vi "ShortcutToFile.vi"(8 "error in (no error)":errorcluster, 10 "write? (F)":bool, 11 "Shortcut file":path) -> (0 "error out":errorcluster, 2 "succeeded?":bool, 3 "Shortcut file out":path)   [LabVIEW 2015]
doc: "This will return a list of items in a folder that are shortcuts (*.lnk). The Path to the Shortcut and the path to item pointed to by the Shortcut are included.\n\nExample:\n Location of Shortcuts: C:\\My Documents\\Misc\n\n Output:\n PATH TO SHORCUT: C:\\My Documents\\Misc\\RF Gain.doc.lnk\n PATH TO ITEM: I:\\Engineers\\John Smith\\RF Gain.doc\n\n PATH TO SHORCUT: C:\\My Documents\\Misc\\Schedule.mpp.lnk\n PATH TO ITEM: I:\\Projects\\ATE\\Planning\\Schedule.mpp\n\n\nReferences:\n Windows Shell - http://msdn.microsoft.com/en-us/library/bb773177(v=VS.85).aspx\n Shell Object - http://msdn.microsoft.com/en-us/library/bb774094(v=VS.85).aspx\n ShellLinkObject Object - http://msdn.microsoft.com/en-us/library/bb774004(v=VS.85).aspx\n\n Changing the icon of EXE files programatically - http://social.msdn.microsoft.com/forums/en-US/csharpgeneral/thread/9e23a82c-8bed-4b96-8b9a-4c2b6136a622/"
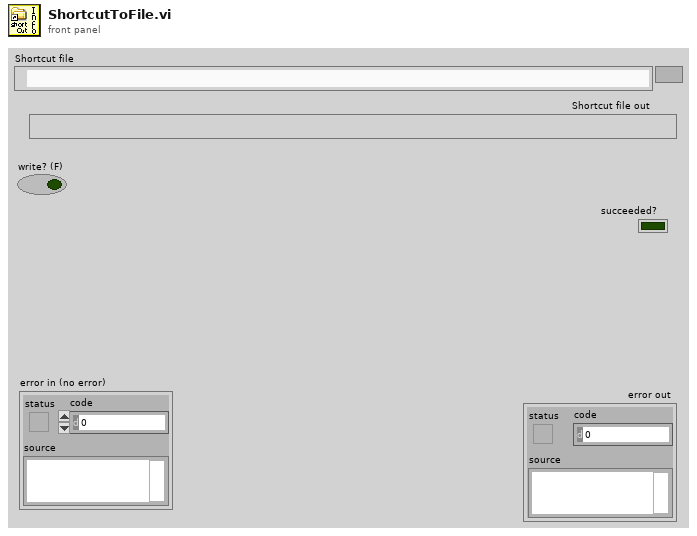
[diagram p1: front panel]
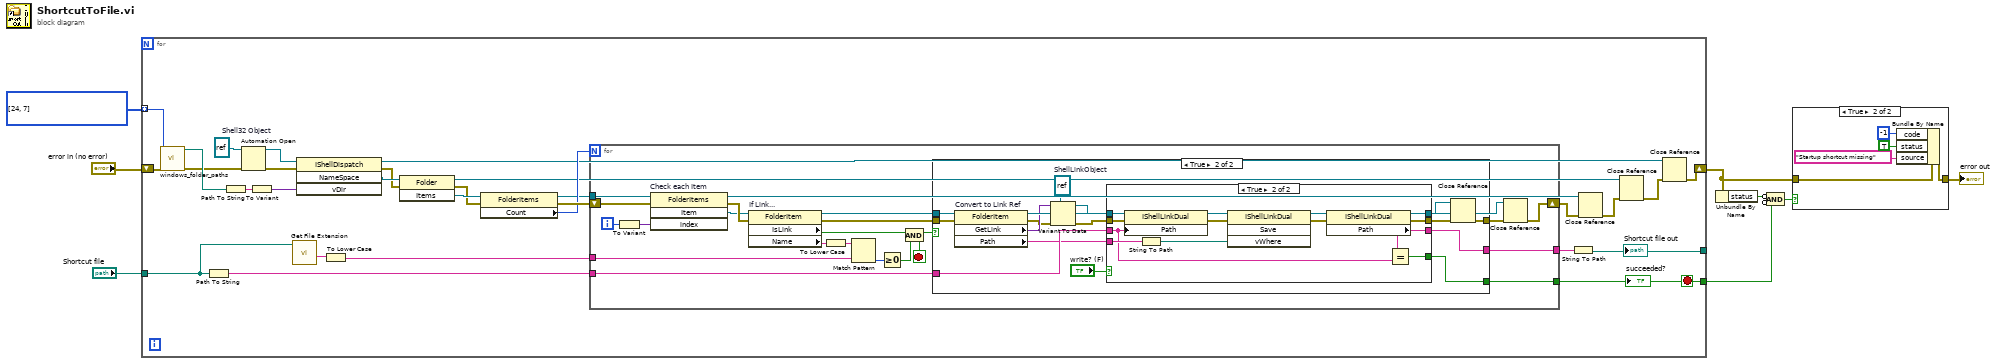
[diagram p0: block diagram]
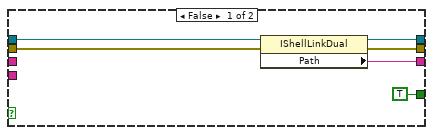
[diagram p3: hidden frame]
diagram:
  n1 = for {
    tunnel: "Shortcut file" -> [w11]
    tunnel: [w12] -> w4
    tunnel: [w36] -> _
    shift-right: [w37] -> w6
    shift-left: "error in (no error)" -> [w14]
    tunnel: i32[] [24, 7] -> [w13] mode=indexing
    stop <- w12 stop-if-true
    w32 = refnum<k7> refnum  # Shell32 Object
    n2 = call "windows_folder_paths.vi"("error in (no error)"=w14, "Folder Role"=w13) -> ("error out"=w15:errorcluster, "System Folder Path"=w16:path)  [unwired: 7 in, 1 out]
    n3 = Path To String(path=w11) -> (string=w18:string)
    n4 = Path To String(path=w16) -> (string=w35:string)
    n5 = Automation Open(error in (no error)=w15, Automation Refnum=w32) -> (Automation Refnum=w31:refnum<k7>, error out=w30:errorcluster)  [unwired: 2 in]
    n6 = To Variant(anything=w35) -> (Variant=w34:variant)
    n7 = call <vilib>:"Get File Extension.vi"("file"=w11) -> ("filename without extension"=w10:string)  [unwired: 6 in, 4 out]
    n8 = invoke on="Get a Ref to the Root Folder" class="IShellDispatch" method="NameSpace"(reference=w31, error in=w30, "vDir"=w34) -> (reference out=w20:refnum<k7>, error out=w27:errorcluster, "NameSpace"=w33:refnum<k7>)  [unwired: 1 in, 1 out]
    n9 = To Lower Case(string=w10) -> (all lower case string=w9:string)
    n10 = invoke class="Folder" method="Items"(reference=w33, error in=w27) -> (reference out=w22:refnum<k7>, error out=w26:errorcluster, "Items"=w28:refnum<k7>)  [unwired: 1 in]
    n11 = property class="FolderItems"(reference=w28, error in=w26) -> (reference out=w24:refnum<k7>, error out=w29:errorcluster, "Count"=w25:i32)
    n12 = for {
      N: w25 -> [_]
      tunnel: w24 -> [w57]
      shift-right: [w42] -> w23
      shift-left: w29 -> [w55]
      tunnel: [w45] -> w17
      tunnel: w18 -> [w41]
      tunnel: [w40] -> w12
      tunnel: w9 -> [w38]
      i -> [w54]
      stop <- w46 stop-if-true
      n13 = To Variant(anything=w54) -> (Variant=w56:variant)
      n14 = invoke on="Check each Item" class="FolderItems" method="Item"(reference=w57, error in=w55, "index"=w56) -> (error out=w53:errorcluster, "Item"=w51:refnum<k7>)  [unwired: 1 in, 2 out]
      n15 = property on="If Link..." class="FolderItem"(reference=w51, error in=w53) -> (reference out=w43:refnum<k7>, error out=w52:errorcluster, "IsLink"=w50:bool, "Name"=w39:string)
      n16 = To Lower Case(string=w39) -> (all lower case string=w49:string)
      n17 = Match Pattern(string=w49, regular expression=w38) -> (offset past match=w48:i32)  [unwired: 1 in, 3 out]
      n18 = Greater Or Equal To 0?(x=w48) -> (x >= 0?=w47:bool)
      n19 = Compound Arithmetic op=AND(w50, w47) -> (w46:bool)
      n20 = case shown="True" w46 {
        tunnel: w52 -> [w58 w68]
        tunnel: w43 -> [_ w70]
        tunnel: [w58 w66] -> w44
        tunnel: [_ w69] -> w45
        tunnel: w41 -> [_ w63]
        tunnel: [_ w59] -> w40
        frame False {
        }
        frame True {
          w71 = refnum<k7> refnum  # ShellLinkObject
          n21 = property on="Convert to Link Ref" class="FolderItem"(reference=w70, error in=w68) -> (error out=w72:errorcluster, "GetLink"=w73:variant, "Path"=w60:string)  [unwired: 1 out]
          n22 = Variant To Data(error in=w72, type=w71, Variant=w73) -> (data=w61:refnum<k7>, error out=w67:errorcluster)
          n23 = case shown="True" "write? (F)" {
            tunnel: w61 -> [w79 w89]
            tunnel: [w75 w82] -> w69
            tunnel: w67 -> [w78 w90]
            tunnel: [w76 w92] -> w65
            tunnel: [w77 w91] -> w64
            tunnel: w63 -> [_ w81]
            tunnel: w60 -> [_ w84]
            tunnel: [TRUE w80] -> w59
            frame False {
              n24 = property class="IShellLinkDual"(reference=w79, error in=w78) -> (reference out=w77:refnum<k7>, error out=w76:errorcluster, "Path"=w75:string)
            }
            frame True {
              n25 = property class="IShellLinkDual"(reference=w89, error in=w90, "Path"=w81) -> (reference out=w88:refnum<k7>, error out=w85:errorcluster)
              n26 = String To Path(string=w84) -> (path=w83:path)
              n27 = invoke class="IShellLinkDual" method="Save"(reference=w88, error in=w85, "vWhere"=w83) -> (reference out=w87:refnum<k7>, error out=w86:errorcluster)  [unwired: 1 in, 2 out]
              n28 = property class="IShellLinkDual"(reference=w87, error in=w86) -> (reference out=w91:refnum<k7>, error out=w92:errorcluster, "Path"=w82:string)
              n29 = Equal?(x=w82, y=w81) -> (x = y?=w80:bool)
            }
          }
          n30 = Close Reference(reference=w64, error in (no error)=w65) -> (error out=w66:errorcluster)
        }
      }
      n31 = Close Reference(reference=w43, error in (no error)=w44) -> (error out=w42:errorcluster)
    }
    "succeeded?" <- w12
    n32 = String To Path(string=w17) -> (path=w36:path)
    "Shortcut file out" <- w36
    n33 = Close Reference(reference=w24, error in (no error)=w23) -> (error out=w21:errorcluster)
    n34 = Close Reference(reference=w22, error in (no error)=w21) -> (error out=w19:errorcluster)
    n35 = Close Reference(reference=w20, error in (no error)=w19) -> (error out=w37:errorcluster)
  }
  n36 = Unbundle By Name(w6) -> ("status"=w5:bool)
  n37 = Compound Arithmetic op=AND(invert w5, invert w4) -> (w3:bool)
  n38 = case shown="True" w3 {
    tunnel: w6 -> [w93 w98]
    tunnel: [w93 w96] -> w7
    frame False {
    }
    frame True {
      n39 = Bundle By Name(cluster=w98, "code"=-1, "status"=TRUE, "source"="Startup shortcut missing" ("error message (\"\")")) -> (w96:errorcluster)
    }
  }
  "error out" <- w7
